vi "main_loop_calculation.vi"(0 "DAQ Data":waveform(dbl)[](array[waveform]), 1 "Offset Parameters":T1={"Separator \nTemperature"=0.0, "Separator Pressure"=0.0, "Upper Dev Section\nTemperature"=0.0, "Upper Dev Section\nPressure"=0.0, "Vapor Tank\nTemperature Offset"=0.0, "Vapor Tank\nPressure "=0.0, "Test Section\nTemperature"=0.0, "Test Section\nPressure"=0.0, "Vapor Inlet \nTemperature"=0.0, "Vapor Inlet\nPressure"=0.0, "Liquid Tank\nTemperature"=0.0, "Liquid Tank\nPressure"=0.0, "Liquid Inlet\nTemperature "=0.0, "Liquid Inlet\nPressure"=0.0, "Atmospheric Pressure [Pa]"=101325.0, "Lower Dev Section\nPressure"=0.0}) -> (2 "Vapor Flow Data":T3, 3 "Liquid Flow Data":T2, 4 "Pressure/Temperature/Mixture Properties":T4)   [LabVIEW 2016]
uses:
  Sensor Translation/sensor_translation.lvlib
  Sensor Translation/Pressure Transducers/Omega/omega_px303_050a5v.vi
  Sensor Translation/Pressure Transducers/Omega/omega_px209_060a5v.vi
  Sensor Translation/MicroFlow Transducers/microflow_mass_flow.vi
  Sensor Translation/MicroFlow Transducers/microflow_density.vi
  Sensor Translation/pressure_unit_converter.vi
  pressure_temp_mixture.ctl
  offset_parameters.ctl
panel:
  out "Separator Temp":dbl
  out "Liquid Inlet T":dbl
  out "Vapor Inlet T Sat":dbl
  # "Saturation\nPressure [Pa]"
  # "Saturation\nTemperature [C]"
  # "Pressure [Pa]"
  # "Temperature [C]"
  # "Liquid Tank"
  # "Separator"
  # "Liquid Inlet"
  # "Vapor Tank"
  # "Vapor Inlet"
  # "Test Section"
  # "Upper Dev Section"
  # "Lower Dev Section"
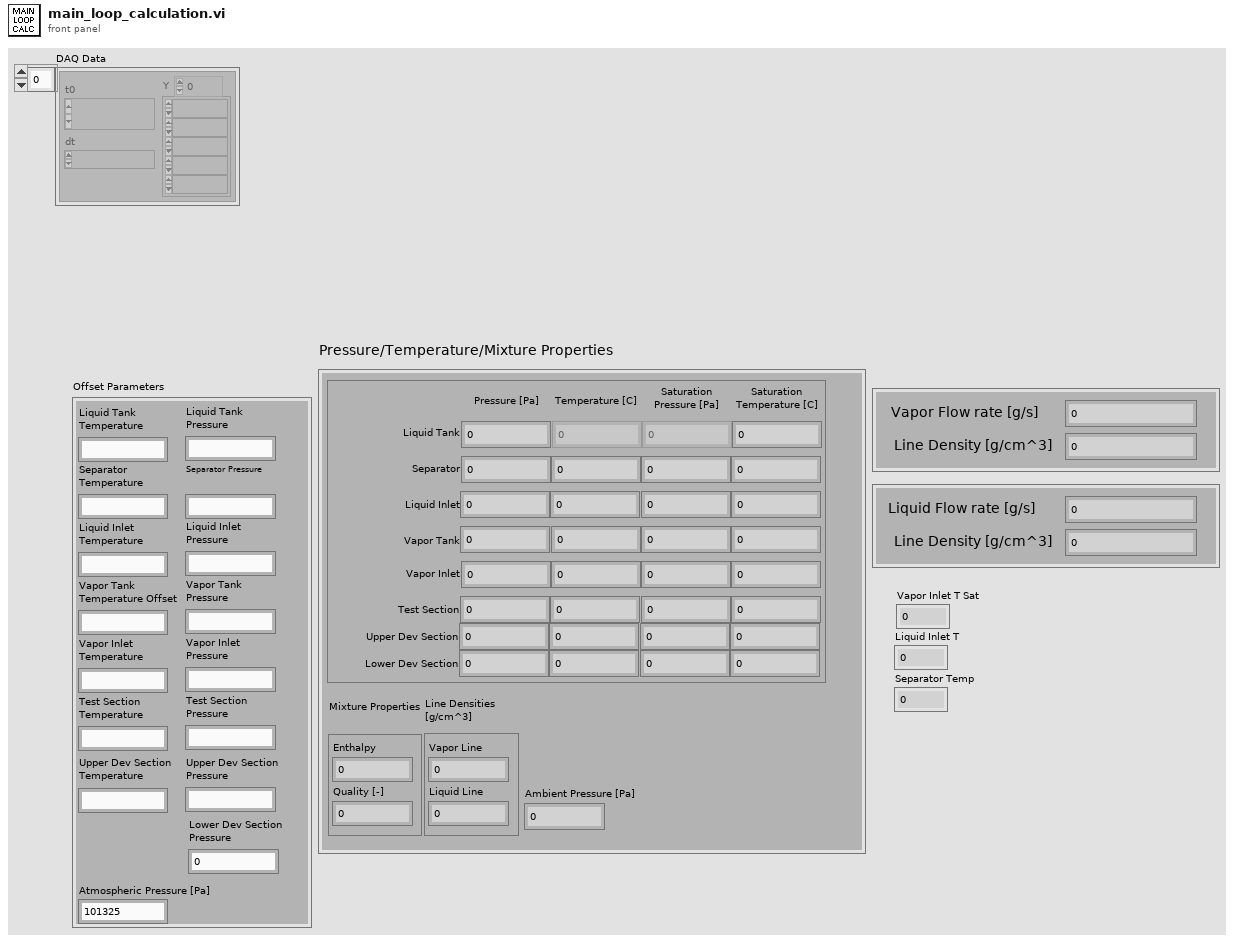
[diagram p1: front panel]
types:
  T1 = typedef "offset_parameters.ctl" = cluster{"Separator \nTemperature":dbl, "Separator Pressure":dbl, "Upper Dev Section\nTemperature":dbl, "Upper Dev Section\nPressure":dbl, "Vapor Tank\nTemperature Offset":dbl, "Vapor Tank\nPressure ":dbl, "Test Section\nTemperature":dbl, "Test Section\nPressure":dbl, "Vapor Inlet \nTemperature":dbl, "Vapor Inlet\nPressure":dbl, "Liquid Tank\nTemperature":dbl, "Liquid Tank\nPressure":dbl, "Liquid Inlet\nTemperature ":dbl, "Liquid Inlet\nPressure":dbl, "Atmospheric Pressure [Pa]":dbl, "Lower Dev Section\nPressure":dbl}
  T2 = cluster{"Liquid Flow rate [g/s]":dbl, "Line Density [g/cm^3]":dbl}
  T3 = cluster{"Vapor Flow rate [g/s]":dbl, "Line Density [g/cm^3]":dbl}
  T4 = typedef "pressure_temp_mixture.ctl" = cluster{"Line Densities\n[g/cm^3]":cluster{"Vapor Line":dbl, "Liquid Line":dbl}, "Mixture Properties":cluster{"Enthalpy":dbl, "Quality [-]":dbl}, "[Readings]":cluster{"Liquid Tank P":dbl, "Liquid Tank T":dbl, "Liquid Tank Sat P":dbl, "Liquid Tank Sat T":dbl, "Separator P":dbl, "Separator T":dbl, "Separator Sat P":dbl, "Separator Sat T":dbl, "Liquid Inlet P":dbl, "Liquid Inlet T":dbl, "Liquid Inlet Sat P":dbl, "Liquid Inlet Sat T":dbl, "Vapor Tank P":dbl, "Vapor Tank T":dbl, "Vapor Tank Sat P":dbl, "Vapor Tank Sat T":dbl, "Vapor Inlet P":dbl, "Vapor Inlet T":dbl, "Vapor Inlet Sat P":dbl, "Vapor Inlet Sat T":dbl, "Test Section P":dbl, "Test Section T":dbl, "Test Section Sat P":dbl, "Test Section Sat T":dbl, "Upper Dev Section P":dbl, "Upper Dev Section T":dbl, "Upper Dev Section Sat P":dbl, "Upper Dev Section Sat T":dbl, "Lower Dev Section P":dbl, "Test Section T 3":dbl, "Lower Dev Section Sat P":dbl, "Lower Dev Section Sat T":dbl}, "Ambient Pressure [Pa]":dbl}
  T5 = cluster{"Rounded Value":dbl, "Rounded Value":dbl}
  T6 = cluster{"mixture enthalpy":dbl, "Quality [-]":dbl}
  T7 = cluster{"array[0]":dbl, "array[1]":dbl, "array[2]":dbl, "array[3]":dbl, "array[4]":dbl, "array[5]":dbl, "array[6]":dbl, "array[7]":dbl, "array[8]":dbl, "array[9]":dbl, "array[10]":dbl, "array[11]":dbl, "array[12]":dbl, "array[13]":dbl, "array[14]":dbl, "array[15]":dbl, "array[16]":dbl, "array[17]":dbl, "array[18]":dbl, "array[19]":dbl, "array[20]":dbl, "array[21]":dbl, "array[22]":dbl, "array[23]":dbl, "array[24]":dbl, "array[25]":dbl, "array[26]":dbl, "array[27]":dbl, "array[28]":dbl, "array[29]":dbl, "array[30]":dbl, "array[31]":dbl}
  T8 = cluster{cluster{"[0]":dbl, "[1]":dbl}, cluster{"mixture enthalpy":dbl, "Quality [-]":dbl}, "Cluster":cluster{"array[0]":dbl, "array[1]":dbl, "array[2]":dbl, "array[3]":dbl, "array[4]":dbl, "array[5]":dbl, "array[6]":dbl, "array[7]":dbl, "array[8]":dbl, "array[9]":dbl, "array[10]":dbl, "array[11]":dbl, "array[12]":dbl, "array[13]":dbl, "array[14]":dbl, "array[15]":dbl, "array[16]":dbl, "array[17]":dbl, "array[18]":dbl, "array[19]":dbl, "array[20]":dbl, "array[21]":dbl, "array[22]":dbl, "array[23]":dbl, "array[24]":dbl, "array[25]":dbl, "array[26]":dbl, "array[27]":dbl, "array[28]":dbl, "array[29]":dbl, "array[30]":dbl, "array[31]":dbl}, "Offset Average":dbl}
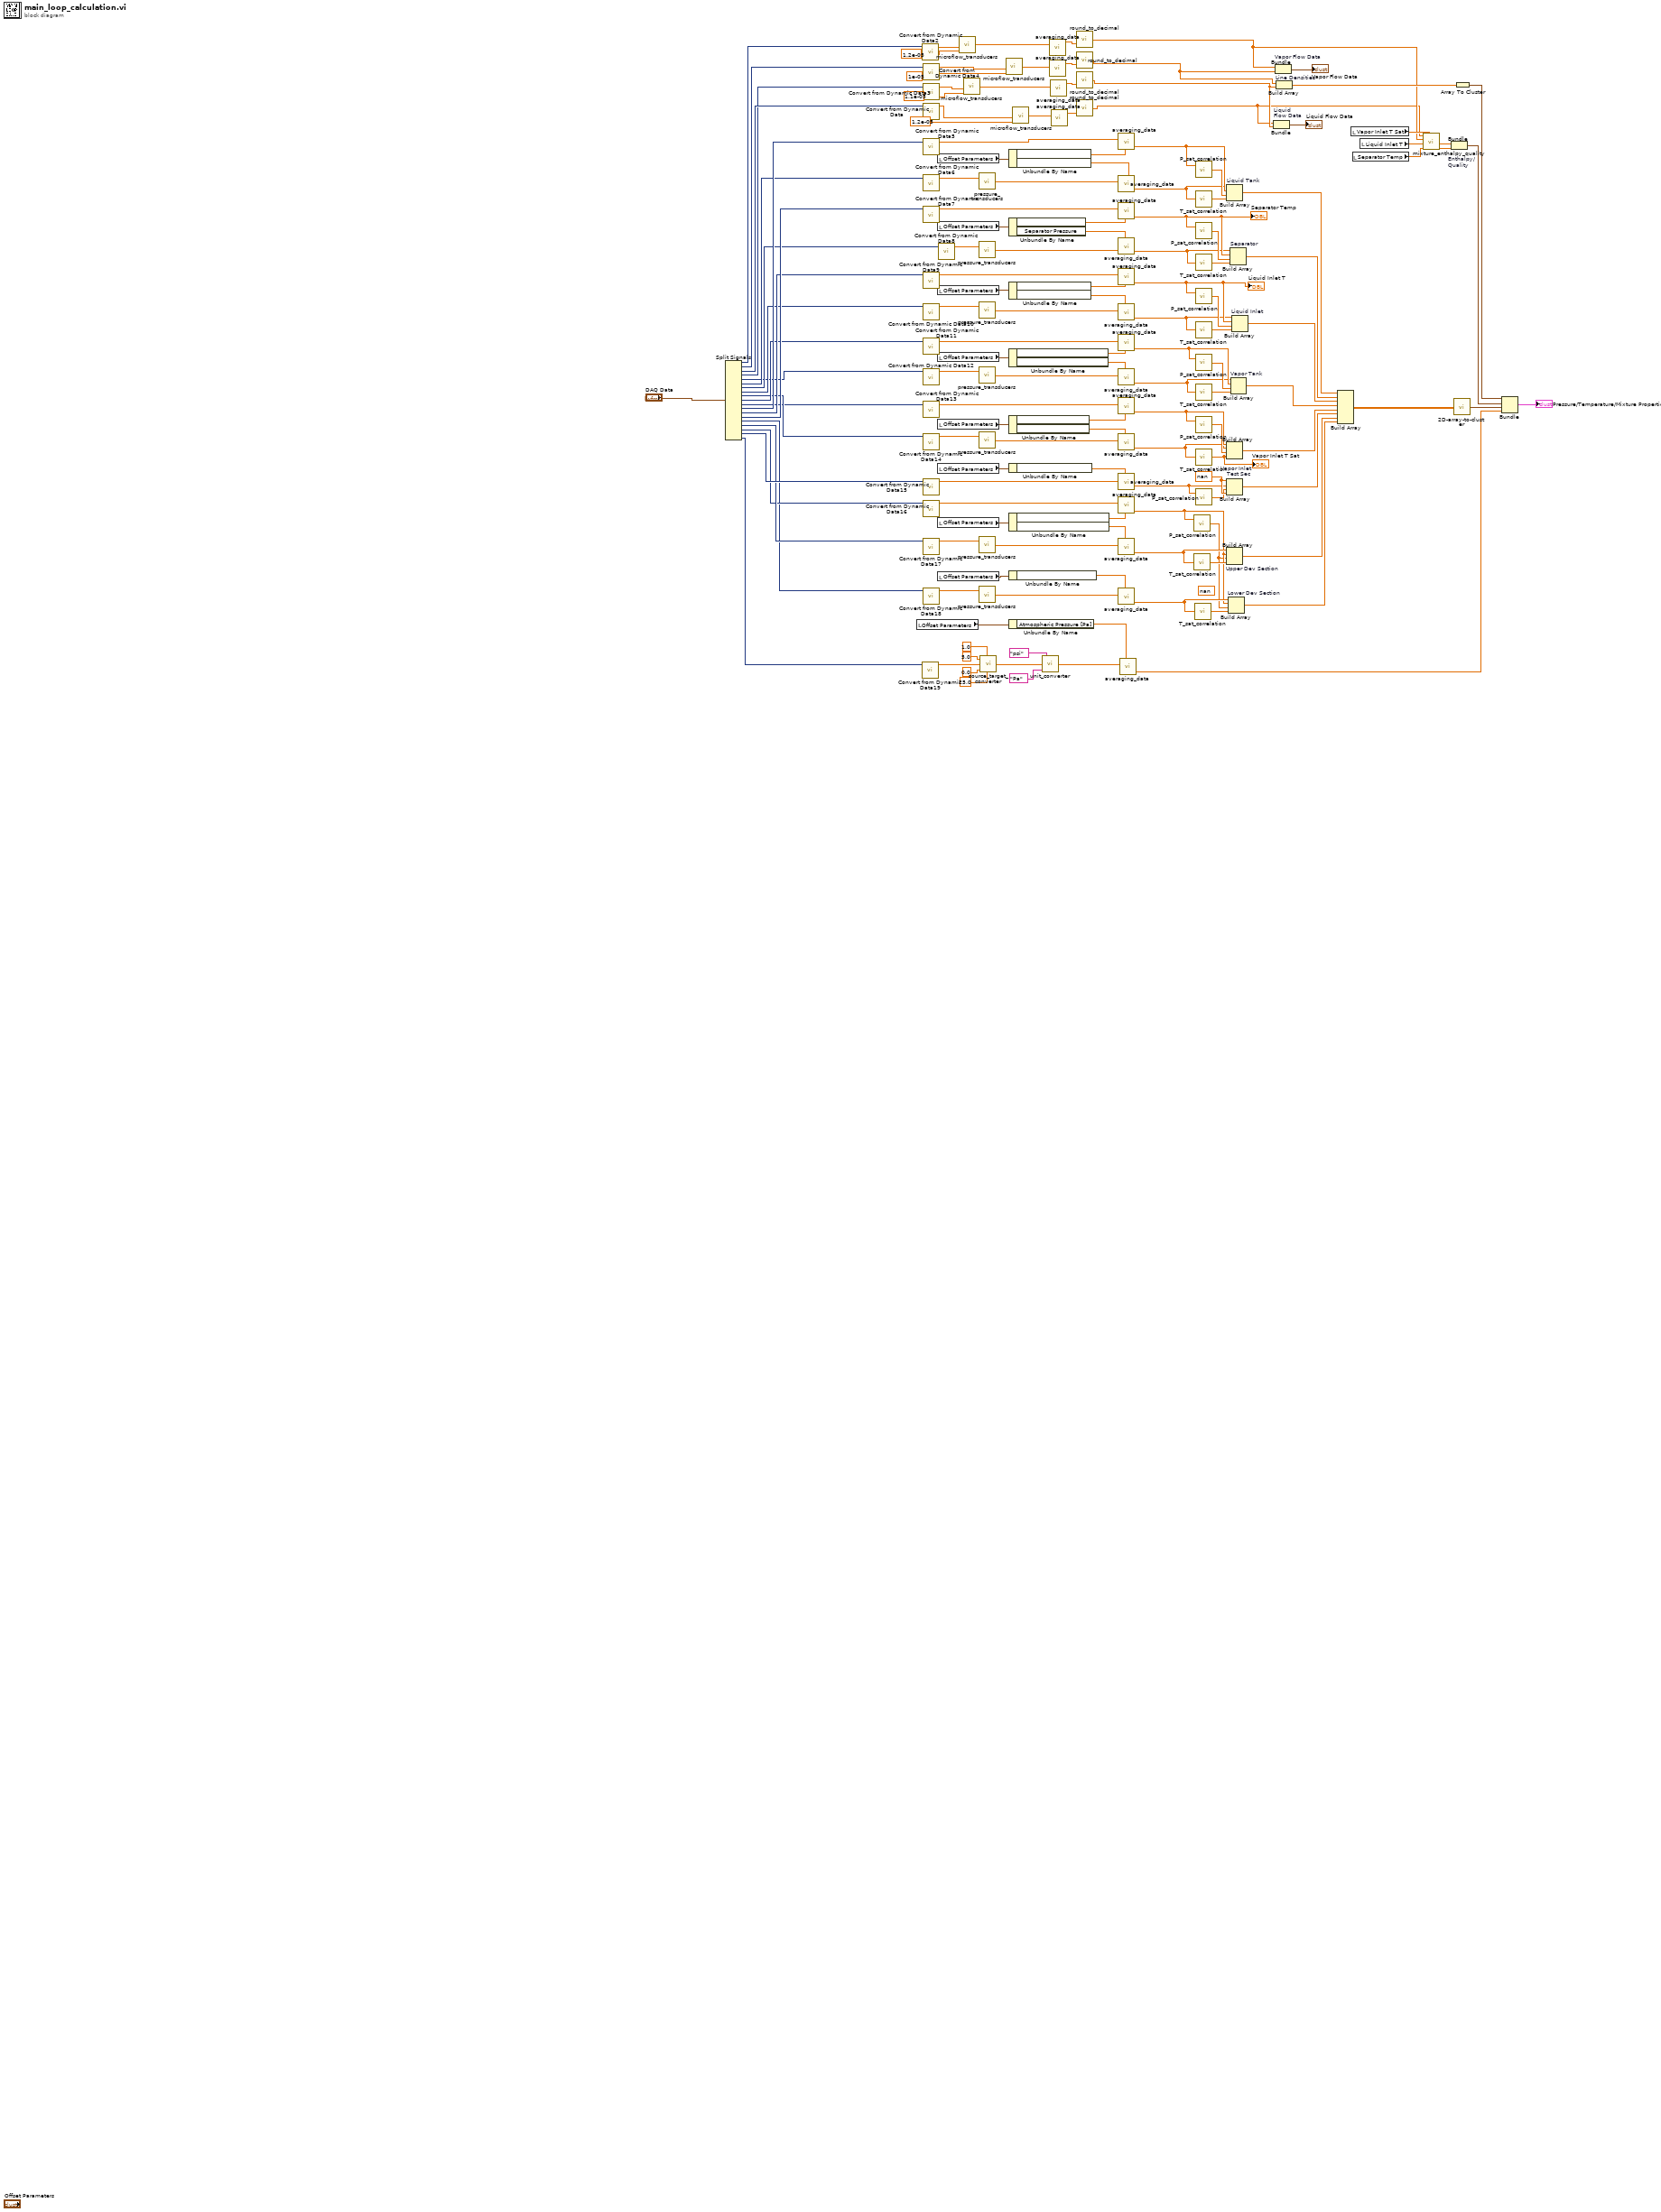
[diagram p0: block diagram]
diagram:
  (unwired) nan ("element")
  w57 = nan ("element")
  n1 = Split Signals("DAQ Data") -> (w122:dynamicdata, w116:dynamicdata, w145:dynamicdata, w144:dynamicdata, w76:dynamicdata, w103:dynamicdata, w95:dynamicdata, w85:dynamicdata, w68:dynamicdata, w78:dynamicdata, w45:dynamicdata, w106:dynamicdata, w90:dynamicdata, w97:dynamicdata, w48:dynamicdata, w51:dynamicdata, w50:dynamicdata, w61:dynamicdata, w12:dynamicdata)  [unwired: 19 in]
  n2 = local read "Offset Parameters"() -> (w124:T1)
  n3 = call "Convert from Dynamic Data19"("Dynamic Data Type"=w12) -> ("Array"=w11:dbl[])  [unwired: 3 in]
  n4 = call "Convert from Dynamic Data2"("Dynamic Data Type"=w122) -> ("Array"=w26:dbl[])  [unwired: 3 in]
  n5 = call "Convert from Dynamic Data4"("Dynamic Data Type"=w116) -> ("Array"=w32:dbl[])  [unwired: 3 in]
  n6 = call "Convert from Dynamic Data3"("Dynamic Data Type"=w144) -> ("Array"=w31:dbl[])  [unwired: 3 in]
  n7 = call "Convert from Dynamic Data"("Dynamic Data Type"=w145) -> ("Array"=w30:dbl[])  [unwired: 3 in]
  n8 = call "Convert from Dynamic Data5"("Dynamic Data Type"=w106) -> ("Array"=w105:dbl[])  [unwired: 3 in]
  n9 = call "Convert from Dynamic Data6"("Dynamic Data Type"=w103) -> ("Array"=w102:dbl[])  [unwired: 3 in]
  n10 = call "Convert from Dynamic Data7"("Dynamic Data Type"=w97) -> ("Array"=w96:dbl[])  [unwired: 3 in]
  n11 = call "Convert from Dynamic Data9"("Dynamic Data Type"=w90) -> ("Array"=w89:dbl[])  [unwired: 3 in]
  n12 = call "Convert from Dynamic Data10"("Dynamic Data Type"=w85) -> ("Array"=w84:dbl[])  [unwired: 3 in]
  n13 = call "Convert from Dynamic Data11"("Dynamic Data Type"=w78) -> ("Array"=w79:dbl[])  [unwired: 3 in]
  n14 = call "Convert from Dynamic Data12"("Dynamic Data Type"=w76) -> ("Array"=w75:dbl[])  [unwired: 3 in]
  n15 = call "Convert from Dynamic Data13"("Dynamic Data Type"=w45) -> ("Array"=w70:dbl[])  [unwired: 3 in]
  n16 = call "Convert from Dynamic Data14"("Dynamic Data Type"=w68) -> ("Array"=w67:dbl[])  [unwired: 3 in]
  n17 = call "Convert from Dynamic Data15"("Dynamic Data Type"=w61) -> ("Array"=w60:dbl[])  [unwired: 3 in]
  n18 = call "Convert from Dynamic Data16"("Dynamic Data Type"=w50) -> ("Array"=w49:dbl[])  [unwired: 3 in]
  n19 = call "Convert from Dynamic Data17"("Dynamic Data Type"=w51) -> ("Array"=w54:dbl[])  [unwired: 3 in]
  n20 = call "Convert from Dynamic Data18"("Dynamic Data Type"=w48) -> ("Array"=w47:dbl[])  [unwired: 3 in]
  n21 = local read "Offset Parameters"() -> (w134:T1)
  n22 = local read "Offset Parameters"() -> (w132:T1)
  n23 = local read "Offset Parameters"() -> (w131:T1)
  n24 = local read "Offset Parameters"() -> (w135:T1)
  n25 = local read "Offset Parameters"() -> (w133:T1)
  n26 = local read "Offset Parameters"() -> (w59:T1)
  n27 = local read "Offset Parameters"() -> (w52:T1)
  n28 = local read "Offset Parameters"() -> (w42:T1)
  n29 = call "Convert from Dynamic Data8"("Dynamic Data Type"=w95) -> ("Array"=w87:dbl[])  [unwired: 3 in]
  n30 = call-poly "microflow_transducers.vi"("Source Offset"=1.2e-05, "Source"=w26) -> ("Target"=w25:dbl[])  [unwired: 2 in]
  n31 = call-poly "microflow_transducers.vi"("Source Offset"=1.1e-05, "Source"=w31) -> ("Target"=w27:dbl[])  [unwired: 2 in]
  n32 = call-poly "pressure_transducers.vi"("Source"=w102) -> ("Target"=w99:dbl[])  [unwired: 1 in]
  n33 = call-poly "pressure_transducers.vi"("Source"=w87) -> ("Target"=w86:dbl[])  [unwired: 1 in]
  n34 = call-poly "pressure_transducers.vi"("Source"=w84) -> ("Target"=w83:dbl[])  [unwired: 1 in]
  n35 = call-poly "pressure_transducers.vi"("Source"=w75) -> ("Target"=w74:dbl[])  [unwired: 1 in]
  n36 = call-poly "pressure_transducers.vi"("Source"=w67) -> ("Target"=w65:dbl[])  [unwired: 1 in]
  n37 = call-poly "pressure_transducers.vi"("Source"=w54) -> ("Target"=w56:dbl[])  [unwired: 1 in]
  n38 = call-poly "pressure_transducers.vi"("Source"=w47) -> ("Target"=w46:dbl[])  [unwired: 1 in]
  n39 = call "source_target_converter.vi"("Source High"=5.0, "Source Low"=1.0, "Source"=w11, "Target Low"=0.0, "Target High"=25.0) -> ("Target"=w4:dbl[])
  n40 = call-poly "microflow_transducers.vi"("Source Offset"=1e-05, "Source"=w32) -> ("Target"=w29:dbl[])  [unwired: 2 in]
  n41 = Unbundle By Name(w134) -> ("Liquid Tank\nTemperature"=w104:dbl, "Liquid Tank\nPressure"=w101:dbl)
  n42 = Unbundle By Name(w132) -> ("Separator \nTemperature"=w98:dbl, "Separator Pressure"=w94:dbl)
  n43 = Unbundle By Name(w131) -> ("Liquid Inlet\nTemperature"=w88:dbl, "Liquid Inlet\nPressure"=w82:dbl)
  n44 = Unbundle By Name(w135) -> ("Vapor Tank\nTemperature Offset"=w77:dbl, "Vapor Tank\nPressure"=w73:dbl)
  n45 = Unbundle By Name(w133) -> ("Vapor Inlet \nTemperature"=w69:dbl, "Vapor Inlet\nPressure"=w66:dbl)
  n46 = Unbundle By Name(w59) -> ("Test Section\nTemperature"=w58:dbl)
  n47 = Unbundle By Name(w52) -> ("Upper Dev Section\nTemperature"=w53:dbl, "Upper Dev Section\nPressure"=w55:dbl)
  n48 = Unbundle By Name(w42) -> ("Lower Dev Section\nPressure"=w41:dbl)
  n49 = Unbundle By Name(w124) -> ("Atmospheric Pressure [Pa]"=w10:dbl)
  n50 = call-poly "microflow_transducers.vi"("Source Offset"=1.2e-05, "Source"=w30) -> ("Target"=w28:dbl[])  [unwired: 2 in]
  n51 = call-poly "unit_converter.vi"("Output Unit"="Pa", "Input"=w4, "Input Unit"="psi") -> ("Output"=w1:dbl[])
  n52 = call "averaging_data.vi"("Input"=w25) -> ("Average"=w19:dbl)  [unwired: 5 in, 2 out]
  n53 = call "averaging_data.vi"("Input"=w29) -> ("Average"=w17:dbl)  [unwired: 5 in, 2 out]
  n54 = call "averaging_data.vi"("Input"=w27) -> ("Average"=w15:dbl)  [unwired: 5 in, 2 out]
  n55 = call "averaging_data.vi"("Input"=w28) -> ("Average"=w13:dbl)  [unwired: 5 in, 2 out]
  n56 = call "round_to_decimal.vi"("Value to Round"=w19) -> ("Rounded Value"=w20:dbl)  [unwired: 1 in]
  n57 = call "round_to_decimal.vi"("Value to Round"=w17) -> ("Rounded Value"=w18:dbl)  [unwired: 1 in]
  n58 = call "round_to_decimal.vi"("Value to Round"=w15) -> ("Rounded Value"=w16:dbl)  [unwired: 1 in]
  n59 = call "round_to_decimal.vi"("Value to Round"=w13) -> ("Rounded Value"=w14:dbl)  [unwired: 1 in]
  n60 = call "averaging_data.vi"("Offset"=w104, "Input"=w105) -> ("Offset Average"=w107:dbl)  [unwired: 4 in, 2 out]
  n61 = call "averaging_data.vi"("Offset"=w101, "Input"=w99) -> ("Offset Average"=w100:dbl)  [unwired: 4 in, 2 out]
  n62 = call "averaging_data.vi"("Offset"=w98, "Input"=w96) -> ("Offset Average"=w93:dbl)  [unwired: 4 in, 2 out]
  "Separator Temp" <- w93
  n63 = call "averaging_data.vi"("Offset"=w94, "Input"=w86) -> ("Offset Average"=w91:dbl)  [unwired: 4 in, 2 out]
  n64 = call "averaging_data.vi"("Offset"=w88, "Input"=w89) -> ("Offset Average"=w81:dbl)  [unwired: 4 in, 2 out]
  "Liquid Inlet T" <- w81
  n65 = call "averaging_data.vi"("Offset"=w82, "Input"=w83) -> ("Offset Average"=w80:dbl)  [unwired: 4 in, 2 out]
  n66 = call "averaging_data.vi"("Offset"=w77, "Input"=w79) -> ("Offset Average"=w72:dbl)  [unwired: 4 in, 2 out]
  n67 = call "averaging_data.vi"("Offset"=w73, "Input"=w74) -> ("Offset Average"=w71:dbl)  [unwired: 4 in, 2 out]
  n68 = call "averaging_data.vi"("Offset"=w69, "Input"=w70) -> ("Offset Average"=w62:dbl)  [unwired: 4 in, 2 out]
  n69 = call "averaging_data.vi"("Offset"=w66, "Input"=w65) -> ("Offset Average"=w64:dbl)  [unwired: 4 in, 2 out]
  n70 = call "averaging_data.vi"("Offset"=w58, "Input"=w60) -> ("Offset Average"=w43:dbl)  [unwired: 4 in, 2 out]
  n71 = call "averaging_data.vi"("Offset"=w53, "Input"=w49) -> ("Offset Average"=w34:dbl)  [unwired: 4 in, 2 out]
  n72 = call "averaging_data.vi"("Offset"=w55, "Input"=w56) -> ("Offset Average"=w40:dbl)  [unwired: 4 in, 2 out]
  n73 = call "averaging_data.vi"("Offset"=w41, "Input"=w46) -> ("Offset Average"=w37:dbl)  [unwired: 4 in, 2 out]
  n74 = call "averaging_data.vi"("Offset"=w10, "Input"=w1) -> ("Offset Average"=w5:dbl)  [unwired: 4 in, 2 out]
  n75 = call "P_sat_correlation.vi"("Temperature"=w34) -> ("P Sat"=w33:dbl)  [unwired: 1 in]
  n76 = call "T_sat_correlation.vi"("P [Pa]"=w40) -> ("T Sat [C]"=w39:dbl)
  n77 = call "T_sat_correlation.vi"("P [Pa]"=w37) -> ("T Sat [C]"=w38:dbl)
  n78 = call "P_sat_correlation.vi"("Temperature"=w107) -> ("P Sat"=w143:dbl)  [unwired: 1 in]
  n79 = call "T_sat_correlation.vi"("P [Pa]"=w100) -> ("T Sat [C]"=w142:dbl)
  n80 = call "P_sat_correlation.vi"("Temperature"=w93) -> ("P Sat"=w136:dbl)  [unwired: 1 in]
  n81 = call "T_sat_correlation.vi"("P [Pa]"=w91) -> ("T Sat [C]"=w92:dbl)
  n82 = call "P_sat_correlation.vi"("Temperature"=w81) -> ("P Sat"=w138:dbl)  [unwired: 1 in]
  n83 = call "T_sat_correlation.vi"("P [Pa]"=w80) -> ("T Sat [C]"=w137:dbl)
  n84 = call "P_sat_correlation.vi"("Temperature"=w72) -> ("P Sat"=w140:dbl)  [unwired: 1 in]
  n85 = call "T_sat_correlation.vi"("P [Pa]"=w71) -> ("T Sat [C]"=w141:dbl)
  n86 = call "P_sat_correlation.vi"("Temperature"=w62) -> ("P Sat"=w139:dbl)  [unwired: 1 in]
  n87 = call "T_sat_correlation.vi"("P [Pa]"=w64) -> ("T Sat [C]"=w63:dbl)
  "Vapor Inlet T Sat" <- w63
  n88 = call "P_sat_correlation.vi"("Temperature"=w43) -> ("P Sat"=w44:dbl)  [unwired: 1 in]
  n89 = Build Array "Liquid Tank"(w100, w107, w143, w142) -> (w126:dbl[])
  n90 = Build Array "Vapor Inlet"(w64, w62, w139, w63) -> (w128:dbl[])
  n91 = Build Array "Test Sec"(w57, w43, w44, w57) -> (w127:dbl[])
  n92 = Build Array "Upper Dev Section"(w40, w34, w33, w39) -> (w36:dbl[])
  n93 = Build Array "Lower Dev Section"(w37, w34, w33, w38) -> (w35:dbl[])
  n94 = Build Array "Separator"(w91, w93, w136, w92) -> (w125:dbl[])
  n95 = Build Array "Vapor Tank"(w71, w72, w140, w141) -> (w129:dbl[])
  n96 = Build Array "Liquid Inlet"(w80, w81, w138, w137) -> (w130:dbl[])
  n97 = Bundle "Liquid\nFlow Data"("Rounded Value"=w14, "Rounded Value"=w16) -> (→"Liquid Flow Data":T5)  [unwired: 1 in]
  n98 = Bundle "Vapor Flow Data"("Rounded Value"=w20, "Rounded Value"=w18) -> (→"Vapor Flow Data":T5)  [unwired: 1 in]
  n99 = Build Array "Line Densities"(w18, w16) -> (w119:dbl[])
  n100 = Build Array(w126, w125, w130, w129, w128, w127, w36, w35) -> (w123:dbl[][])
  n101 = local read "Vapor Inlet T Sat"() -> (w110:dbl)
  n102 = local read "Separator Temp"() -> (w112:dbl)
  n103 = local read "Liquid Inlet T"() -> (w111:dbl)
  n104 = call "mixture_enthalpy_quality.vi"("Vapor Inlet Pressure [Pa]"=w110, "Separator Temp [C]"=w112, "Liquid Inlet Temp [C]"=w111, "Vapor Flow Rate [g/s]"=w20, "Liquid Flow Rate [g/s]"=w14) -> ("Quality [-]"=w120:dbl, "mixture enthalpy"=w121:dbl)  [unwired: 2 out]
  n105 = Bundle "Enthalpy/\nQuality"("mixture enthalpy"=w121, "Quality [-]"=w120) -> (w114:T6)  [unwired: 1 in]
  n106 = call "2D-array-to-cluster.vi"("2D Array"=w123) -> ("Cluster"=w115:T7)
  n107 = Array To Cluster(array=w119) -> (cluster=w113:cluster{"[0]":dbl, "[1]":dbl})
  n108 = Bundle(w113, w114, "Cluster"=w115, "Offset Average"=w5) -> (→"Pressure/Temperature/Mixture Properties":T8)  [unwired: 1 in]
